vi "TBQ_ComputeStatistics.vi"(11 "TimeBasedQueue In":refnum<class "TimeBasedQueue.lvclass">) -> (0 "Standard Deviation":dbl format="%0.2f", 1 "Mean":dbl format="%0.2f", 3 "TimeBasedQueue Out":refnum<class "TimeBasedQueue.lvclass">)   [LabVIEW 2012, in "TimeBasedQueue.lvclass"]
uses:
  TimeBasedQueue.lvclass
  TimeBasedQueue.lvclass/TimeBasedQueue.ctl
  <vilib>/Analysis/NI_AALBase.lvlib
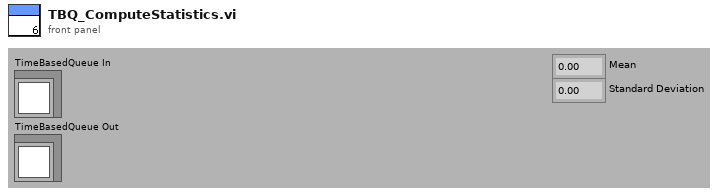
[diagram p1: front panel]
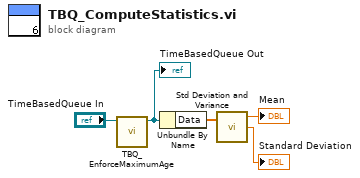
[diagram p0: block diagram]
diagram:
  n1 = call "TBQ_EnforceMaximumAge.vi"("TimeBasedQueue In"="TimeBasedQueue In") -> ("TimeBasedQueue Out"=w3:refnum<class "TimeBasedQueue.lvclass">)  [unwired: 10 in]
  "TimeBasedQueue Out" <- w3
  n2 = Unbundle By Name(w3) -> ("Data"=w4:dbl[])
  n3 = call <vilib>:"Std Deviation and Variance.vi"("X"=w4) -> ("mean"=→"Mean":dbl, "standard deviation"=→"Standard Deviation":dbl)  [unwired: 1 in, 1 out]
